vi "NGTS_DAQmx AO Write Data.vi"(5 "timeout":dbl=0.05, 8 "error  in":errorcluster, 10 "AO Data for Tasks":cluster{"AO Setpoints":dbl[]}[](array[cluster]), 11 "AO Tasks In":refnum<k21>[](array[refnum])) -> (0 "error out":errorcluster, 3 "AO Tasks Out":refnum<k21>[](array[refnum]))   [LabVIEW 2018]
uses:
  <vilib>/DAQmx/write.llb/DAQmx Write (Analog 1D DBL NChan 1Samp).vi
  <vilib>/DAQmx/miscellaneous.llb/DAQmx Fill In Error Info.vi
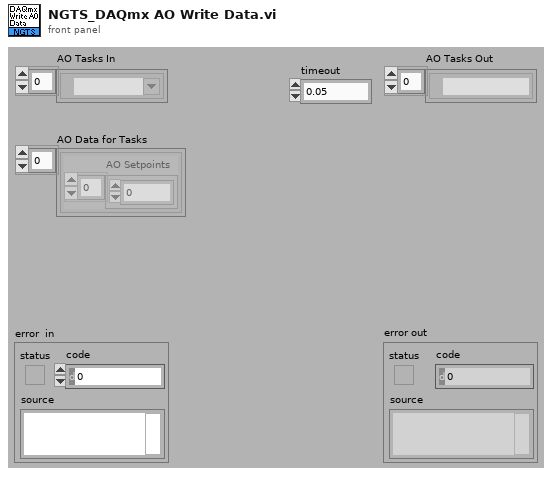
[diagram p1: front panel]
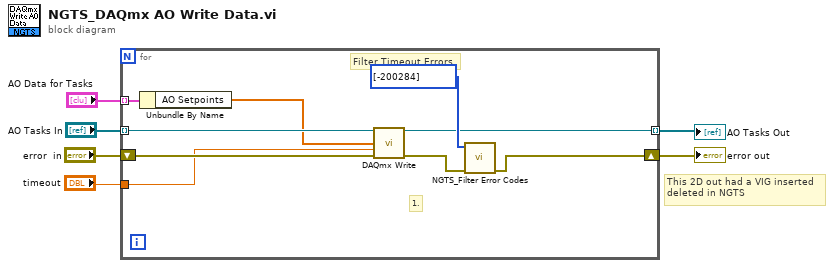
[diagram p0: block diagram]
diagram:
  # "This 2D out had a VIG inserted\ndeleted in NGTS"
  n1 = for {
    tunnel: "AO Tasks In" -> [w14] mode=indexing
    shift-right: [w7] -> w2
    shift-left: "error  in" -> [w15]
    tunnel: [w8] -> w5 mode=indexing
    tunnel: "timeout" -> [w11]
    tunnel: "AO Data for Tasks" -> [w10] mode=indexing
    # "Filter Timeout Errors"
    # "1."
    n2 = Unbundle By Name(w10) -> ("AO Setpoints"=w9:dbl[])
    n3 = call-poly <vilib>:"DAQmx Write.vi"("task/channels in"=w14, "data"=w9, "timeout"=w11, "error in"=w15) -> ("task out"=w8:refnum<k21>, "error out"=w13:errorcluster)  [unwired: 9 in, 1 out]
    n4 = call "NGTS_Filter Error Codes.vi"("error in (no error)"=w13, "Filter Error Codes"=i32[] [-200284]) -> ("error out"=w7:errorcluster)  [unwired: 9 in]
  }
  "AO Tasks Out" <- w5
  "error out" <- w2
